vi "Is hostname mDNS.vi"(11 "address":string) -> (3 "mDNS?":bool)   [LabVIEW 2020, in "NI_WFCN.lvlib"]
doc: "Determine if the specified hostname belongs to a mDNS-managed TLD."
uses:
  <vilib>/net/WFCN/NI_WFCN.lvlib
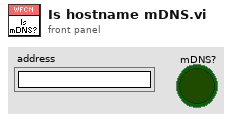
[diagram p1: front panel]
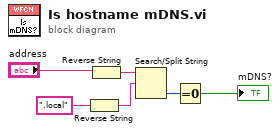
[diagram p0: block diagram]
diagram:
  n1 = Reverse String(1:".local" ("string")) -> (0:w1:string)
  n2 = Reverse String(1:"address") -> (0:w2:string)
  n3 = Search/Split String(string=w2, search string/char (-)=w1) -> (offset of match=w3:i32)  [unwired: 1 in, 2 out]
  n4 = Equal To 0?(x=w3) -> (x = 0?=→"mDNS?":bool)
